vi "Norm[-1;1].vi"(9 "Min":dbl=10.0 format="%#_13g", 10 "Max":dbl=100.0 format="%#_13g", 11 "Original Value":dbl) -> (3 "Norm Value":dbl)   [LabVIEW 2020]
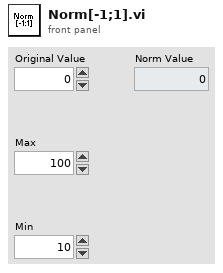
[diagram p1: front panel]
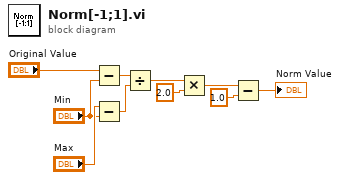
[diagram p0: block diagram]
diagram:
  n1 = Subtract(x="Original Value", y="Min") -> (x-y=w5:dbl)
  n2 = Subtract(x="Max", y="Min") -> (x-y=w6:dbl)
  n3 = Divide(x=w5, y=w6) -> (x/y=w7:dbl)
  n4 = Multiply(x=w7, y=2.0 ("x")) -> (x*y=w9:dbl)
  n5 = Subtract(x=w9, y=1.0) -> (x-y=→"Norm Value":dbl)
